vi "DVR test.vi"() -> ()   [LabVIEW 2010]
uses:
  Classes/Data_Class/Data.lvclass
  Classes/Data_Class/Scalar_Class/Float32_Class/Float32.lvclass
panel:
  out "data value reference":refnum<data-value>
  out "specific class reference":refnum<data-value>
  out "error out 3":errorcluster
  out "error out 2":errorcluster
  out "error out":errorcluster
  out "data value":refnum<class "Data.lvclass">
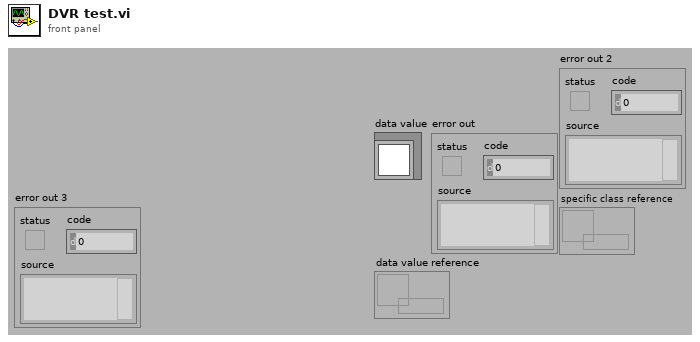
[diagram p1: front panel]
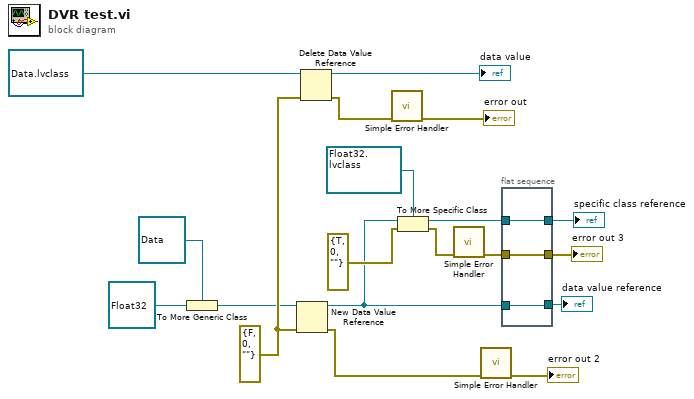
[diagram p0: block diagram]
diagram:
  w18 = errorcluster {"status"=FALSE, "code"=0, "source"=""} ("error in (no error)")
  n1 = To More Generic Class(target class=refnum<class "Data.lvclass"> refnum ("Data.lvclass"), reference=refnum<class "Float32.lvclass"> refnum ("Float32.lvclass")) -> (generic class reference=w8:refnum<class "Data.lvclass">)
  n2 = New Data Value Reference(data value=w8, error in=w18) -> (data value reference=w1:refnum<data-value>, error out=w19:errorcluster)
  n3 = Delete Data Value Reference(data value reference=refnum<data-value> refnum ("data value reference 2"), error in=w18) -> (data value=→"data value":refnum<class "Data.lvclass">, error out=w17:errorcluster)
  n4 = call <vilib>:"Simple Error Handler.vi"("error in (no error)"=w17) -> ("error out"=→"error out":errorcluster)  [unwired: 4 in, 4 out]
  n5 = To More Specific Class(target class=refnum<data-value> refnum ("data value reference"), reference=w1, error in=errorcluster {"status"=TRUE, "code"=0, "source"=""} ("error in (no error)")) -> (specific class reference=w6:refnum<data-value>, error out=w12:errorcluster)
  n6 = call <vilib>:"Simple Error Handler.vi"("error in (no error)"=w12) -> ("error out"=w4:errorcluster)  [unwired: 4 in, 4 out]
  n7 = call <vilib>:"Simple Error Handler.vi"("error in (no error)"=w19) -> ("error out"=→"error out 2":errorcluster)  [unwired: 4 in, 4 out]
  n8 = flat-sequence {
    tunnel: [w22] -> w7
    tunnel: w6 -> [w22]
    tunnel: [w21] -> w5
    tunnel: w4 -> [w21]
    tunnel: [w20] -> w3
    tunnel: w1 -> [w20]
    frame #0 {
    }
  }
  "error out 3" <- w5
  "specific class reference" <- w7
  "data value reference" <- w3
